vi "List Topics.vi"(8 "error in (no error)":errorcluster, 9 "Region":T1, 11 "AWS Credentials":T2) -> (0 "error out":errorcluster, 3 "Topics out":refnum<class "Topic.lvclass">[](array[class]))   [LabVIEW 2015, in "NI_AWS_SNS.lvlib" / "Topic.lvclass"]
doc: "Returns a list of the requester's topics.\n\nThis action is throttled at 30 transactions per second (TPS)."
uses:
  Topic.lvclass
  Core/HTTP Request/AWS Credentials.ctl
  Core/HTTP Request/Region.ctl
  Core/HTTP Request/HTTP Request.lvclass/HTTP Request.ctl
  Core/HTTP Request/Write Credentials.vi
  Core/HTTP Request/Write Region.vi
  Core/HTTP Request/Write Service.vi
  Core/HTTP Request/Write Verify Server.vi
  Core/ARN/ARN.lvclass
  Core/HTTP Request/HTTP Request.lvclass
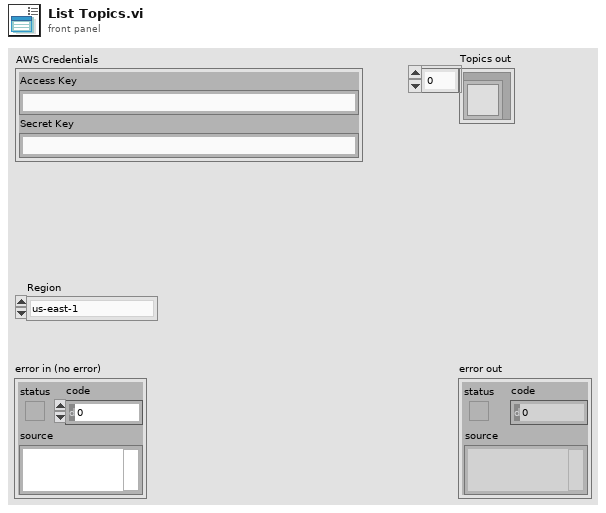
[diagram p1: front panel]
types:
  T1 = typedef "NI_AWS_Core.lvlib/HTTP Request.lvclass/Region.ctl" = enum16{"us-east-1", "us-east-2", "us-west-1", "us-west-2", "ap-northeast-1", "ap-northeast-2", "ap-southeast-1", "ap-southeast-2", "ca-central-1", "eu-central-1", "eu-west-1", "eu-west-2", "sa-east-1"}
  T2 = typedef "NI_AWS_Core.lvlib/HTTP Request.lvclass/AWS Credentials.ctl" = cluster{"Access Key":string, "Secret Key":string}
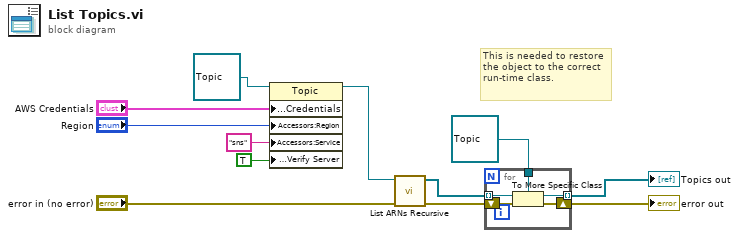
[diagram p0: block diagram]
diagram:
  # "This is needed to restore the object to the correct run-time class."
  n1 = property class="Topic"(reference=refnum<class "Topic.lvclass"> refnum ("NI_AWS_SNS.lvlib:Topic"), "Accessors:Credentials"="AWS Credentials", "Accessors:Region"="Region", "Accessors:Service"="sns" ("Service"), "Accessors:Verify Server"=TRUE ("Verify Server")) -> (reference out=w5:refnum<class "Topic.lvclass">)  [unwired: 1 in, 1 out]
  n2 = call "List ARNs Recursive.vi"("error in (no error)"="error in (no error)", "ARN in"=w5) -> ("error out"=w1:errorcluster, "ARNs out"=w3:refnum<class "ARN.lvclass">[])  [unwired: 8 in]
  n3 = for {
    tunnel: refnum<class "Topic.lvclass"> refnum ("NI_AWS_SNS.lvlib:Topic") -> [w17]
    tunnel: w3 -> [w16] mode=indexing
    tunnel: [w15] -> w11 mode=indexing
    shift-right: [w13] -> w12
    shift-left: w1 -> [w14]
    n4 = To More Specific Class(target class=w17, reference=w16, error in=w14) -> (specific class reference=w15:refnum<class "Topic.lvclass">, error out=w13:errorcluster)
  }
  "error out" <- w12
  "Topics out" <- w11
